vi "CSTK_Enum Creator.vi"   [LabVIEW 2015]
uses:
  Library/Enum Creator/CSTK_Enum Creator.lvlib
panel:
  # "Enum Creator"
types:
  T1 = enum32{"Invalid", "Standard", "Closed", "Hidden", "Minimized", "Maximized"}
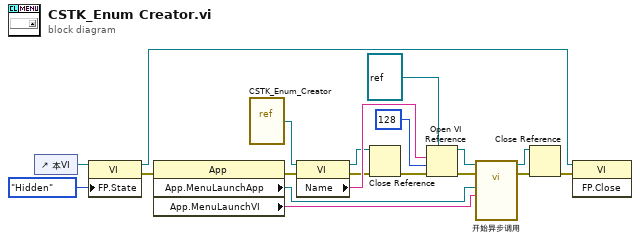
[diagram p0: block diagram]
diagram:
  n1 = control-ref of="本VI"() -> (w18:refnum<vi>)
  n2 = property class="VI"(reference=w18, "FP.State"=T1."Hidden" ("前面板窗口:状态")) -> (reference out=w5:refnum<vi>, error out=w8:errorcluster)  [unwired: 1 in]
  n3 = property class="App"(error in=w8) -> (error out=w7:errorcluster, "App.MenuLaunchApp"=w10:refnum<vi>, "App.MenuLaunchVI"=w9:string)  [unwired: 1 in, 1 out]
  n4 = vi-ref "CSTK_Enum_Creator.vi"() -> (w16:refnum<vi>)
  n5 = property class="VI"(reference=w16, error in=w7) -> (reference out=w3:refnum<vi>, error out=w2:errorcluster, "Name"=w19:string)
  n6 = Close Reference(reference=w3, error in (no error)=w2) -> (error out=w1:errorcluster)
  n7 = Open VI Reference(type specifier VI Refnum (for type only)=refnum<vi> refnum ("类型说明符VI引用句柄（仅用于类型）"), vi path=w19, options=128 ("选项"), error in (no error)=w1) -> (vi reference=w14:refnum<vi>, error out=w13:errorcluster)  [unwired: 2 in]
  n8 = call-by-ref "开始异步调用"(reference=w14, error in=w13, "应用程序:菜单启动:VI"=w9, "应用程序引用（本地）"=w10) -> (reference out=w12:refnum<vi>, error out=w11:errorcluster)  [unwired: 10 in]
  n9 = Close Reference(reference=w12, error in (no error)=w11) -> (error out=w4:errorcluster)
  n10 = invoke class="VI" method="FP.Close"(reference=w5, error in=w4) -> ()  [unwired: 1 in, 3 out]
